vi "Add Tim Eyes.vi"(7 "Options":T1={"Eye Size"=1.0, "Overlay Eyes?"=TRUE, "Eye Tracking?"=TRUE} {"Eye Size" items=["Small"=0.5, "Medium"=1, "Large"=2]}, 8 "error in (no error)":errorcluster, 9 "Eye Coordinates":cluster{"X":sgl, "Y":sgl}[](array[cluster])=[{"X"=125.0, "Y"=67.0}, {"X"=189.0, "Y"=65.0}], 10 "Feature Coordinates":cluster{"Y":sgl, "X":sgl}[](array[cluster]), 11 "ImageRef In":T2=refnum) -> (0 "error out":errorcluster, 3 "ImageRef out":T2)   [LabVIEW 2014]
doc: "This SubVI will overlay some googley eyes onto an image, in accordance to the \"Eye Coordinates\" Input. The pupils of the eye will then look towards the Coordinates of a user defines \"Feature\".\n\nEye Options allow you to enable/disable and change the size of the Googley Eyes"
uses:
  <vilib>/vision/Image Controls.llb/IMAQ Image.ctl
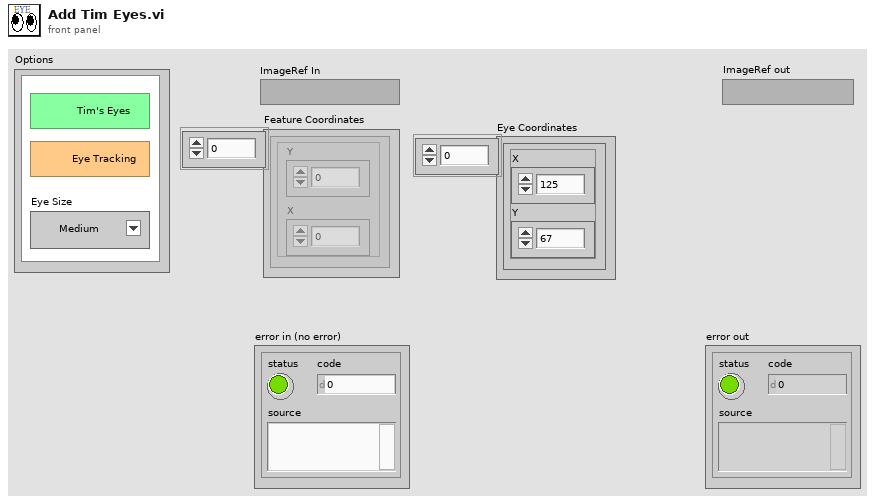
[diagram p1: front panel]
types:
  T1 = cluster{"Eye Size":sgl, "Overlay Eyes?":bool, "Eye Tracking?":bool}
  T2 = typedef "IMAQ Image.ctl" = refnum<image>
  T3 = cluster{"Left":i32, "Top":i32, "Right":i32, "Bottom":i32}
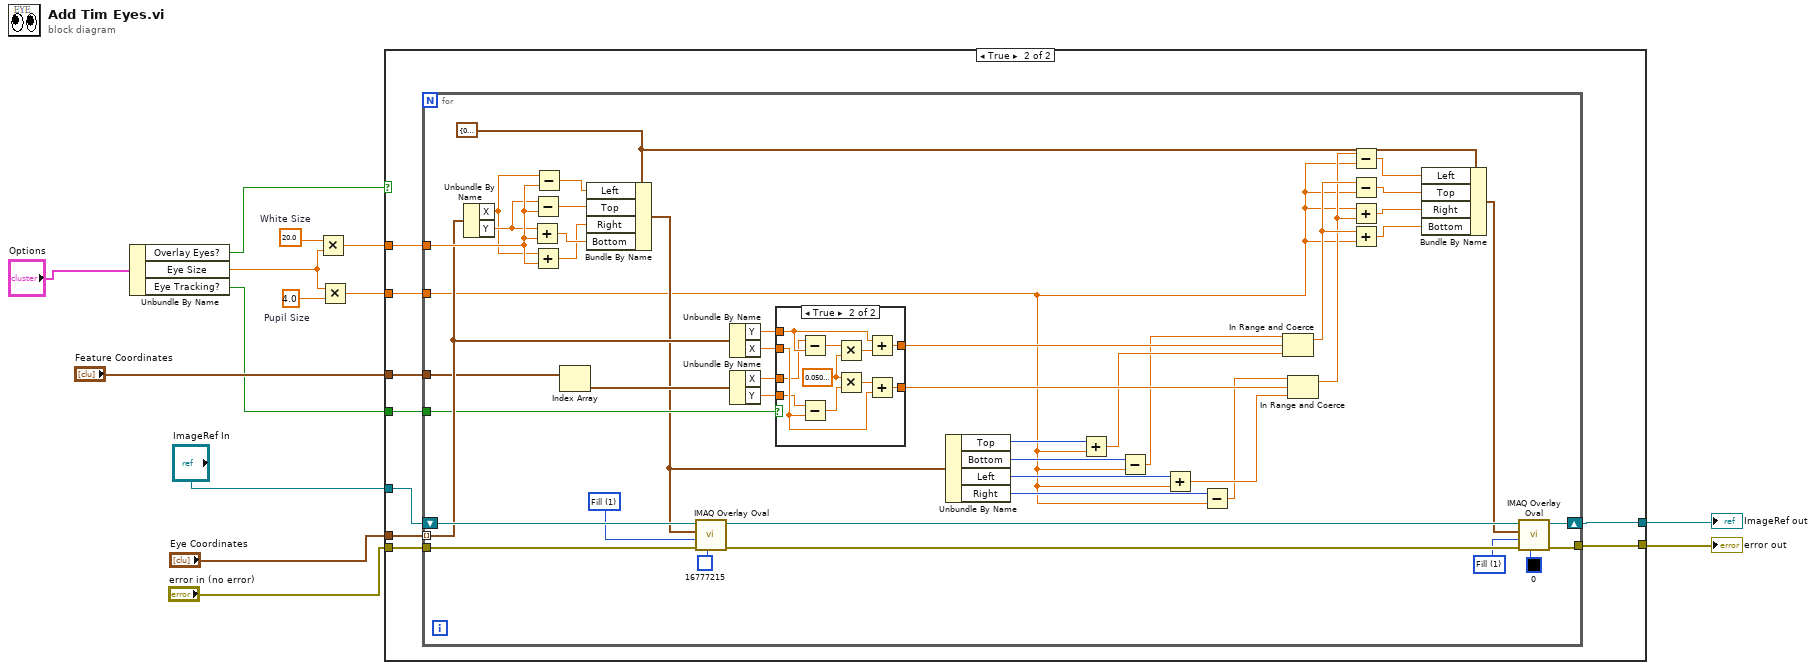
[diagram p0: block diagram]
diagram:
  w10 = sgl 4.0  # Pupil Size
  w11 = sgl 20.0  # White Size
  n1 = Unbundle By Name("Options") -> ("Overlay Eyes?"=w8:bool, "Eye Size"=w5:sgl, "Eye Tracking?"=w3:bool)
  n2 = Multiply(x=w11, y=w5) -> (x*y=w9:sgl)
  n3 = Multiply(x=w5, y=w10) -> (x*y=w6:sgl)
  n4 = case shown="True" w8 {
    tunnel: "error in (no error)" -> [w16 w24]
    tunnel: [w16 w22] -> w12
    tunnel: "Eye Coordinates" -> [_ w21]
    tunnel: [w15 w23] -> w13
    tunnel: "ImageRef In" -> [w15 w25]
    tunnel: w9 -> [_ w20]
    tunnel: w6 -> [_ w19]
    tunnel: "Feature Coordinates" -> [_ w18]
    tunnel: w3 -> [_ w17]
    frame False {
    }
    frame True {
      n5 = for {
        tunnel: w24 -> [w69]
        tunnel: [w64] -> w22
        tunnel: w21 -> [w46] mode=indexing
        shift-right: [w63] -> w23
        shift-left: w25 -> [w70]
        tunnel: w20 -> [w58]
        tunnel: w19 -> [w26]
        tunnel: w18 -> [w45]
        tunnel: w17 -> [w44]
        w59 = u32 1 items=["Frame", "Fill"] ("Drawing Mode (Frame)")
        w67 = u32 1 items=["Frame", "Fill"] ("Drawing Mode (Frame)")
        w61 = T3 {"Left"=0, "Top"=0, "Right"=0, "Bottom"=0} ("Bounding Rectangle")
        n6 = Unbundle By Name(w46) -> ("X"=w56:sgl, "Y"=w57:sgl)
        n7 = Add(x=w57, y=w58) -> (x+y=w39:sgl)
        n8 = Subtract(x=w57, y=w58) -> (x-y=w42:sgl)
        n9 = Add(x=w56, y=w58) -> (x+y=w38:sgl)
        n10 = Subtract(x=w56, y=w58) -> (x-y=w37:sgl)
        n11 = Index Array(array=w45) -> (element=w47:cluster{"Y":sgl, "X":sgl})  [unwired: 1 in]
        n12 = Bundle By Name(cluster=w61, "Left"=w37, "Top"=w42, "Right"=w38, "Bottom"=w39) -> (w35:T3)
        n13 = call "IMAQ Overlay Oval"("Color"=u32 16777215, "error in (no error)"=w69, "Drawing Mode (Frame)"=w67, "Bounding Rectangle"=w35, "Image"=w70) -> ("error out"=w65:errorcluster, "Image Out"=w66:T2)  [unwired: 5 in]
        n14 = Unbundle By Name(w46) -> ("Y"=w50:sgl, "X"=w51:sgl)
        n15 = Unbundle By Name(w47) -> ("X"=w48:sgl, "Y"=w49:sgl)
        n16 = case shown="True" w44 {
          tunnel: w51 -> [w71 w83]
          tunnel: w50 -> [w72 w80]
          tunnel: w49 -> [_ w76]
          tunnel: w48 -> [_ w75]
          tunnel: [w72 w74] -> w43
          tunnel: [w71 w73] -> w40
          frame False {
          }
          frame True {
            w79 = sgl 0.05 ("y")
            n17 = Subtract(x=w75, y=w80) -> (x-y=w77:sgl)
            n18 = Subtract(x=w76, y=w83) -> (x-y=w78:sgl)
            n19 = Multiply(x=w77, y=w79) -> (x*y=w81:sgl)
            n20 = Multiply(x=w79, y=w78) -> (x*y=w82:sgl)
            n21 = Add(x=w80, y=w81) -> (x+y=w74:sgl)
            n22 = Add(x=w82, y=w83) -> (x+y=w73:sgl)
          }
        }
        n23 = Unbundle By Name(w35) -> ("Top"=w34:i32, "Bottom"=w32:i32, "Left"=w30:i32, "Right"=w28:i32)
        n24 = Add(x=w34, y=w26) -> (x+y=w33:sgl)
        n25 = Subtract(x=w32, y=w26) -> (x-y=w31:sgl)
        n26 = Add(x=w30, y=w26) -> (x+y=w29:sgl)
        n27 = Subtract(x=w28, y=w26) -> (x-y=w27:sgl)
        n28 = In Range and Coerce(upper limit=w31, x=w43, lower limit=w33) -> (coerced(x)=w41:sgl)  [unwired: 1 out]
        n29 = In Range and Coerce(upper limit=w27, x=w40, lower limit=w29) -> (coerced(x)=w36:sgl)  [unwired: 1 out]
        n30 = Subtract(x=w36, y=w26) -> (x-y=w53:sgl)
        n31 = Subtract(x=w41, y=w26) -> (x-y=w52:sgl)
        n32 = Add(x=w26, y=w36) -> (x+y=w54:sgl)
        n33 = Add(x=w41, y=w26) -> (x+y=w55:sgl)
        n34 = Bundle By Name(cluster=w61, "Left"=w53, "Top"=w52, "Right"=w54, "Bottom"=w55) -> (w60:T3)
        n35 = call "IMAQ Overlay Oval"("Color"=u32 0, "error in (no error)"=w65, "Drawing Mode (Frame)"=w59, "Bounding Rectangle"=w60, "Image"=w66) -> ("error out"=w64:errorcluster, "Image Out"=w63:T2)  [unwired: 5 in]
      }
    }
  }
  "ImageRef out" <- w13
  "error out" <- w12
